vi "PDF Protokoll Dichtheitstest.vi"(8 "error in (no error)":errorcluster caption="Fehler (Eingang, kein Fehler)") -> (0 "error out":errorcluster caption="Fehler (Ausgang)")   [LabVIEW 2020, in "Erweiterte Konfig.lvlib"]
uses:
  Erweiterte Konfig.lvlib
  Dichtheitstest Umfang.ctl
  System Einstellungen V2/Aktioen FGV System Konstanten.ctl
  Status Dichtheitstest Aktionen.ctl
  FGV PID Aktionen.ctl
  <vilib>/Utility/miscctls.llb/LVPrintingMarginsTypeDef.ctl
  Allgemein/allgemeine Sub-VIs.lvlib
  System Einstellungen V2/System Einstellungen V2.lvlib
panel:
  out "Dichtheitstest Umfang":T1 items=["Pumpe / Filter / FT-IR / PNS", "Pumpe / Filter / FT-IR", "Filter / FT-IR", "FT-IR"]
  out "zul. Druckabfall:":string
  out "Dauer Dichtheitstest:":string
  out "Bestanden":bool caption="Boolesch"
  out "Druckanstieg:":string
  out "Enddruck:":string
  out "Startdruck:":string
  out "Umfang:":string
  out "Endzeit:":string
  out "Startzeit:":string
  out "Ser.Nr.:":string caption="Serien Nummer:"
  out "Messgerät:":string
  # "Dichtheitstest"
  # "mbar"
  # "mbar"
  # "mbar"
  # "IAG-Industrie Automatisierungsgeschellschaft m.b.H.    l  Industriestraße 2    l    2722Weikersdorf     )+43262221734 7+43262221734655"
  # "mbar"
  # "s"
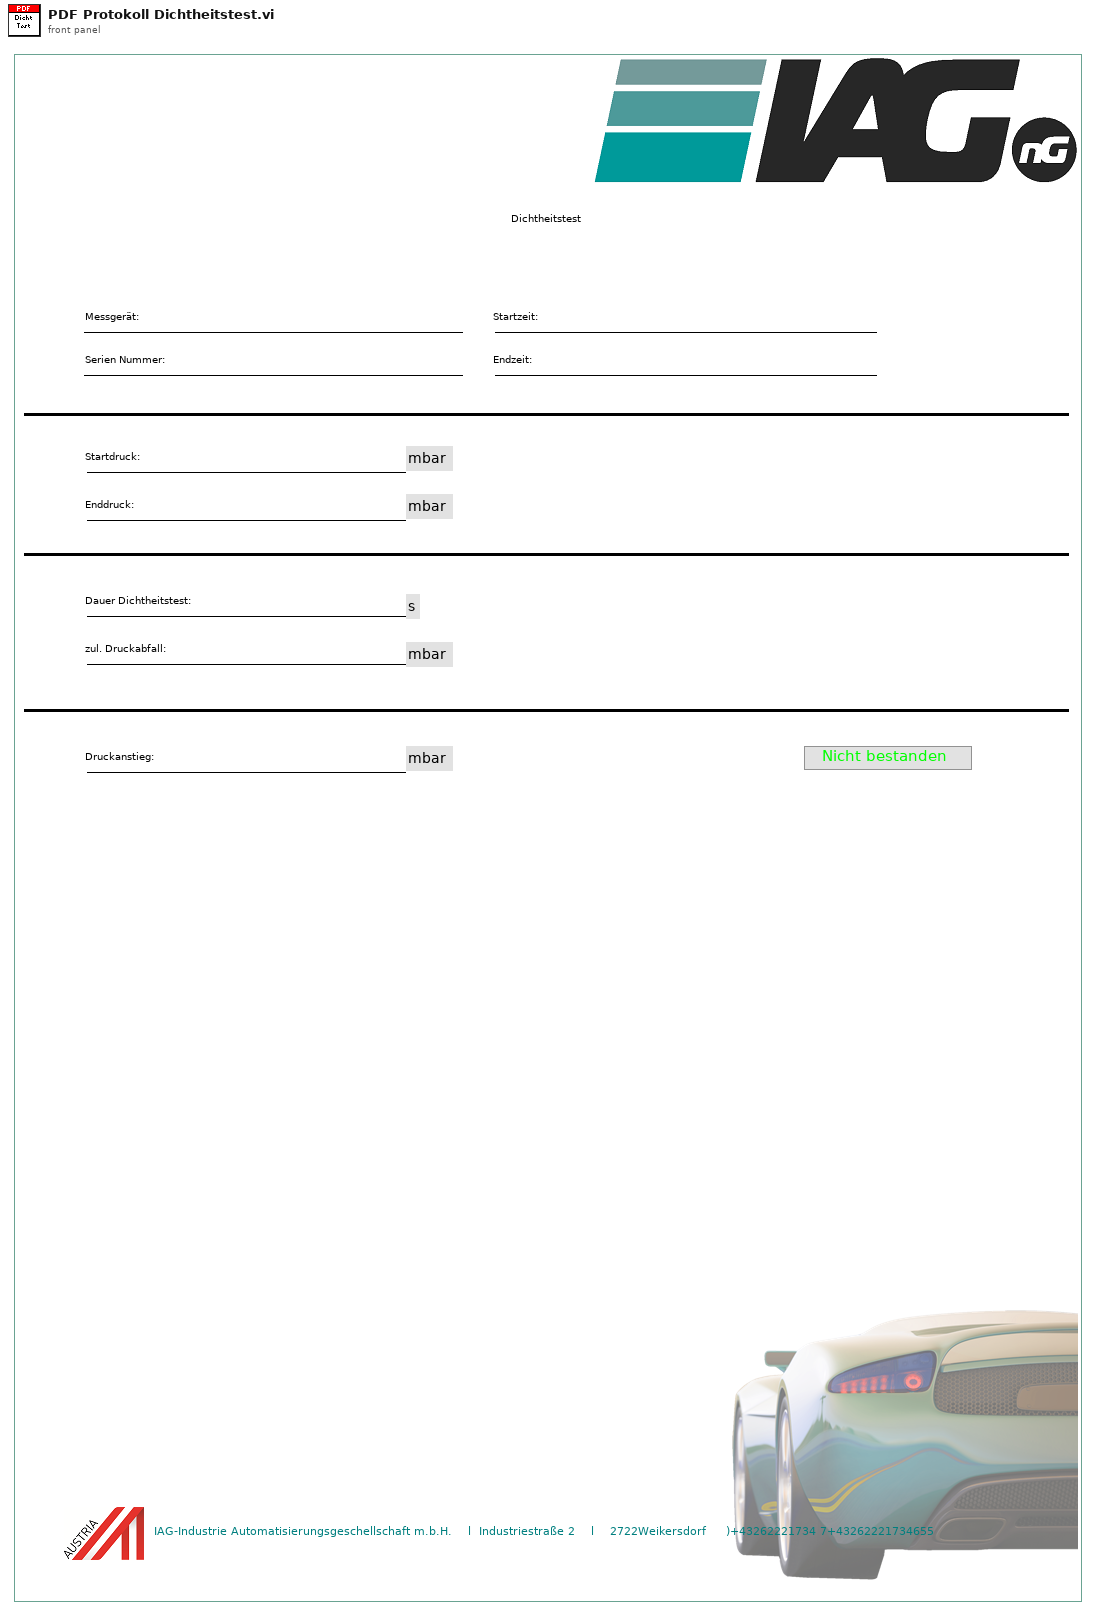
[diagram p1: front panel]
types:
  T1 = typedef "Erweiterte Konfig.lvlib/Dichtheitstest Umfang.ctl" = u16
  T2 = typedef "Erweiterte Konfig.lvlib/FGV PID Aktionen.ctl" = enum16{"Lesen", "Schreiben PID", "Schreiben Sonstige", "Dichtheitstest", "Aktionen Dicht.", "Parameter Sensor"}
  T3 = typedef "Erweiterte Konfig.lvlib/Status Dichtheitstest Aktionen.ctl" = enum16{"lesen", "Zeitstempel", "Daten", "läuft", "Protokolldaten"}
  T4 = typedef "System Einstellungen V2.lvlib/Aktioen FGV System Konstanten.ctl" = enum16{"lesen", "laden", "speichern", "Sprache"}
  T5 = enum32{"Portrait", "Landscape", "Rotated Portrait", "Rotated Landscape"}
  T6 = typedef "LVPrintingMarginsTypeDef.ctl" = cluster{"Top":sgl, "Left":sgl, "Bottom":sgl, "Right":sgl, "Measurement System":enum8{"Inches", "cm"}}
  T7 = typedef "Erweiterte Konfig.lvlib/Dichtheitstest Protokoll.ctl" = cluster{"Startzeit":timestamp, "Endzeit":timestamp, "Startdruck":sgl, "Enddruck":sgl, "Dichtheitstest Umfang":T1}
  T8 = typedef "Erweiterte Konfig.lvlib/Sonstige Parameter.ctl" = cluster{"Lüfter langsam":sgl, "Lüfter schnell":sgl, "FT-IR Kühlung Soll":sgl, "FT-IR Kühlung Max":sgl, "Überwachung":T9, "Befüllung aktiv":T10, "Stickstoff Befüllzeit":sgl, "Befüllintervall":sgl, "Kalibrierwert FT-IR":sgl, "Offset Ausgang":sgl, "Offset FT-IR":sgl, "Offset Druck FT-IR":sgl, "Dichtheitstest Zeit":sgl, "Dichtheitstest Abfall":sgl, "Dichtheitstest Umfang":T1, "Offset Umgebung":sgl, "Max Taupunkt":sgl, "Pumpendrehzahl":sgl, "ext. Befüllung":T10, "Ext. Stickstoff Befüllzeit":sgl}
  T9 = typedef "Auswahlfeld.ctl" = u16
  T10 = typedef "LogKonfig.lvlib/Auswahlfeld aktiviert-deaktiviert.ctl" = u16
  T11 = cluster{"Modell":string, "ProjektNummer":string, "Software Version":string, "Seriennummer":string}
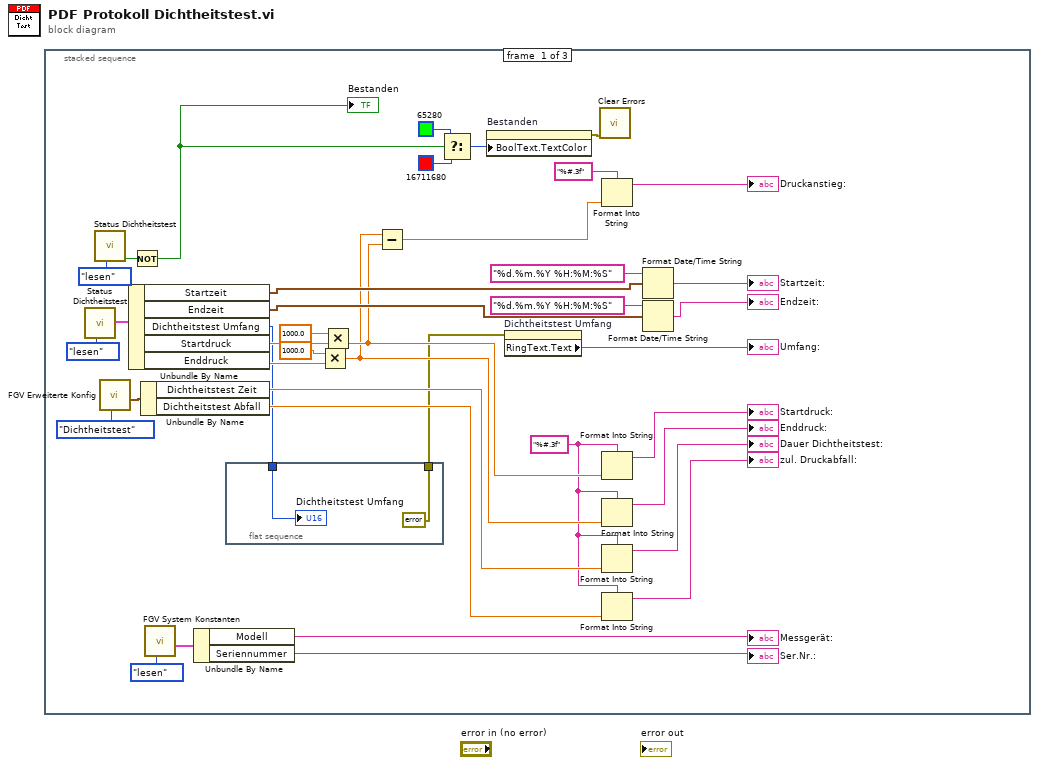
[diagram p0: block diagram]
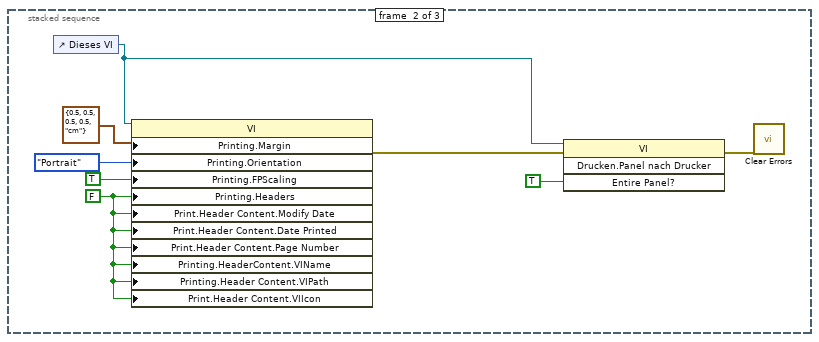
[diagram p2: hidden frame]
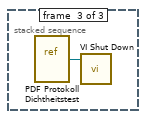
[diagram p3: hidden frame]
diagram:
  n1 = stacked-sequence {
    frame #0 {
      w4 = "%#.3f" ("Format-String")
      n2 = call "Status Dichtheitstest.vi"("Aktionen"=Status_Dichtheitstest_Aktionen."lesen") -> ("Protokoll"=w20:T7)  [unwired: 6 in, 4 out]
      n3 = call "Status Dichtheitstest.vi"("Aktionen"=Status_Dichtheitstest_Aktionen."lesen") -> ("Fehler"=w13:bool)  [unwired: 6 in, 4 out]
      n4 = call "FGV Erweiterte Konfig.vi"("Aktion"=FGV_PID_Aktionen."Dichtheitstest") -> ("Sonstige"=w16:T8)  [unwired: 6 in, 4 out]
      n5 = Unbundle By Name(w20) -> ("Startzeit"=w19:timestamp, "Endzeit"=w18:timestamp, "Dichtheitstest Umfang"=w3:T1, "Startdruck"=w11:sgl, "Enddruck"=w10:sgl)
      n6 = Not(x=w13) -> (.not. x?=w12:bool)
      "Bestanden" <- w12
      n7 = Unbundle By Name(w16) -> ("Dichtheitstest Zeit"=w15:sgl, "Dichtheitstest Abfall"=w14:sgl)
      n8 = call "FGV System Konstanten.vi"("Aktionen"=Aktioen_FGV_System_Konstanten."lesen") -> ("Cluster out"=w39:T11)  [unwired: 6 in, 4 out]
      n9 = Unbundle By Name(w39) -> ("Modell"=→"Messgerät:":string, "Seriennummer"=→"Ser.Nr.:":string)
      n10 = flat-sequence {
        tunnel: w3 -> [w42]
        tunnel: [errorcluster {"status"=FALSE, "code"=0, "source"=""} ("Fehler (Eingang, kein Fehler)")] -> w1
        frame #0 {
          "Dichtheitstest Umfang" <- w42
        }
      }
      n11 = Multiply(x=sgl 1000.0, y=w10) -> (x*y=w7:sgl)
      n12 = Multiply(x=sgl 1000.0, y=w11) -> (x*y=w8:sgl)
      n13 = Subtract(x=w7, y=w8) -> (x-y=w9:sgl)
      n14 = Select(t=u32 65280, s=w12, f=u32 16711680) -> (s? t:f=w24:u32)
      n15 = property on="Bestanden" class="Bool. (strikt)"("BoolText.TextColor"=w24) -> (error out=w23:errorcluster)  [unwired: 2 in, 1 out]
      n16 = property on="Dichtheitstest Umfang" class="Ring (strikt)"(error in=w1) -> ("RingText.Text"=→"Umfang:":string)  [unwired: 1 in, 2 out]
      n17 = call <vilib>:"Clear Errors.vi"("error in (no error)"=w23) -> ()  [unwired: 5 in, 2 out]
      n18 = Format Into String(format string="%#.3f" ("Format-String"), w9) -> (resulting string=→"Druckanstieg:":string)  [unwired: 2 in, 1 out]
      n19 = Format Into String(format string=w4, w8) -> (resulting string=→"Startdruck:":string)  [unwired: 2 in, 1 out]
      n20 = Format Into String(format string=w4, w7) -> (resulting string=→"Enddruck:":string)  [unwired: 2 in, 1 out]
      n21 = Format Into String(format string=w4, w15) -> (resulting string=→"Dauer Dichtheitstest:":string)  [unwired: 2 in, 1 out]
      n22 = Format Into String(format string=w4, w14) -> (resulting string=→"zul. Druckabfall:":string)  [unwired: 2 in, 1 out]
      n23 = Format Date/Time String(time format string (%c)="%d.%m.%Y %H:%M:%S" ("Zeitformatierungs-String (%c)"), seconds (now)=w19) -> (date/time string=→"Startzeit:":string)  [unwired: 1 in]
      n24 = Format Date/Time String(time format string (%c)="%d.%m.%Y %H:%M:%S" ("Zeitformatierungs-String (%c)"), seconds (now)=w18) -> (date/time string=→"Endzeit:":string)  [unwired: 1 in]
    }
    frame #1 {
      w45 = FALSE ("Drucken:Kopfzeilen?")
      n25 = control-ref of="Dieses VI"() -> (w48:refnum<vi>)
      n26 = property class="VI"(reference=w48, "Printing.Margin"=T6 {"Top"=0.5, "Left"=0.5, "Bottom"=0.5, "Right"=0.5, "Measurement System"=enum."cm"} ("Drucken:Ränder"), "Printing.Orientation"=T5."Portrait" ("Drucken:Seitenausrichtung"), "Printing.FPScaling"=TRUE ("Drucken:Frontpanel-Skalierung?"), "Printing.Headers"=w45, "Print.Header Content.Modify Date"=w45, "Print.Header Content.Date Printed"=w45, "Print.Header Content.Page Number"=w45, "Printing.HeaderContent.VIName"=w45, "Printing.Header Content.VIPath"=w45, "Print.Header Content.VIIcon"=w45) -> (error out=w50:errorcluster)  [unwired: 1 in, 1 out]
      n27 = invoke class="VI" method="Drucken.Panel nach Drucker"(reference=w48, error in=w50, "Entire Panel?"=TRUE ("Abschnittskopfzeilen?")) -> (error out=w43:errorcluster)  [unwired: 1 in, 3 out]
      n28 = call <vilib>:"Clear Errors.vi"("error in (no error)"=w43) -> ()  [unwired: 5 in, 2 out]
    }
    frame #2 {
      n29 = vi-ref "PDF Protokoll Dichtheitstest.vi"() -> (w51:refnum<vi>)
      n30 = call "VI Shut Down.vi"("VI Referenz"=w51) -> ()  [unwired: 11 in]
    }
  }
